vi "Find Droplets Freeze Time.vi"(8 "Error In":errorcluster, 10 "GreyLevel Drops and time Derivative in":dbl[][](array[numeric]), 11 "Rel Time Array":u32[](array[numeric])) -> (0 "Error Out":errorcluster, 3 "FreezeYesNo":T1, 4 "DropletBaselineSTD":dbl[](array[numeric]), 6 "DropletBaseline":dbl[](array[numeric]))   [LabVIEW 2013]
uses:
  TypeDef/FreezePointData.ctl
  DB/ConfDB.ctl
  DB/ConfEnum.ctl
  <vilib>/Analysis/NI_AALBase.lvlib
panel:
  out "Numeric":i32
  out "Derivative":cluster{u32[], "GreyLevelArray":dbl[]}[](graph)
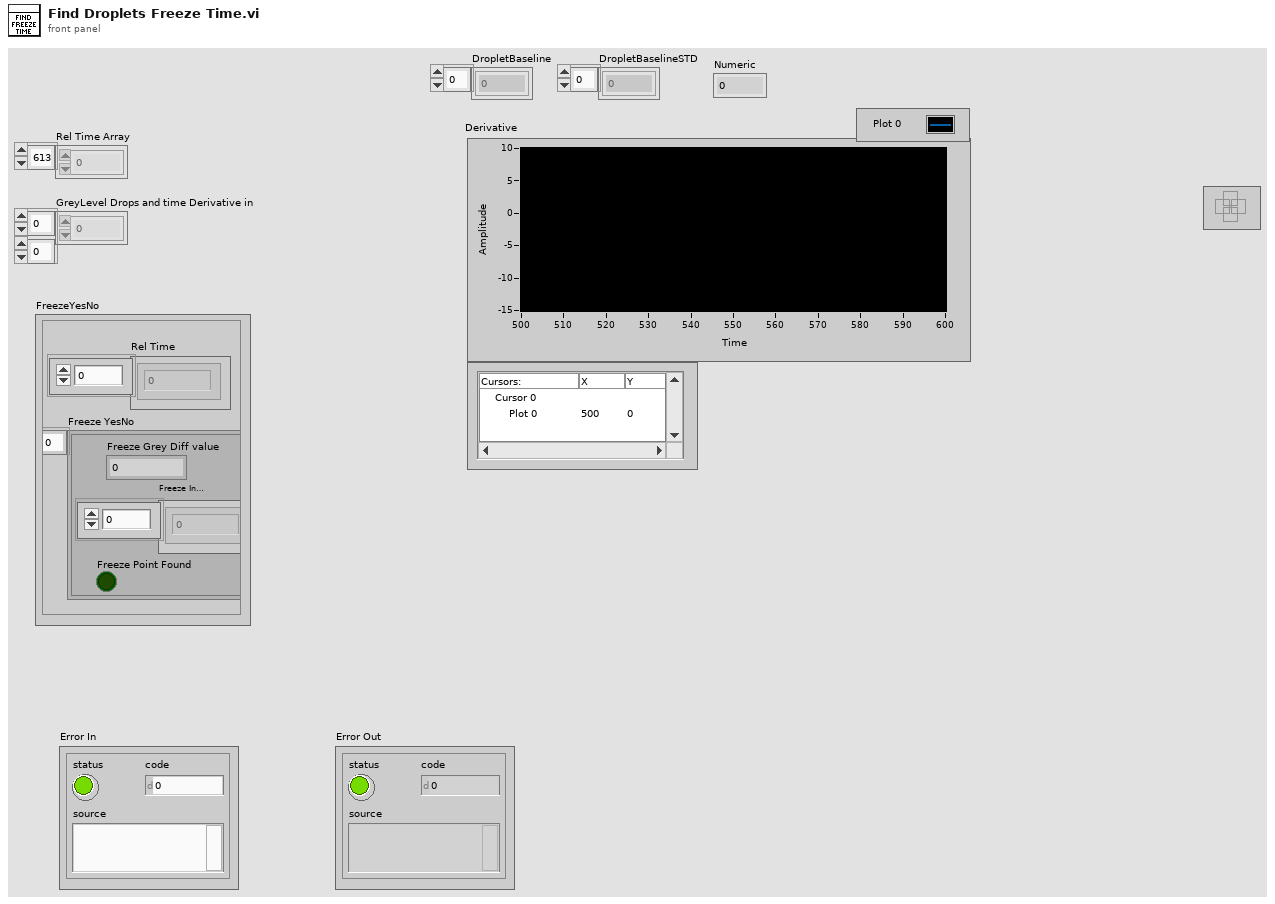
[diagram p1: front panel]
types:
  T1 = typedef "FreezePointData.ctl" = cluster{"Freeze YesNo":cluster{"Freeze Grey Diff value":dbl, "Freeze Point Found":bool, "Freeze Indices":u32[]}[], "Rel Time":u32[]}
  T2 = cluster{"Freeze Grey Diff value":dbl, "Freeze Point Found":bool, "Freeze Indices":u32[]}[]
  T3 = typedef "ConfEnum.ctl" = enum16{"Init", "GetConfDB", "GetTemperatureAtIndex", "WriteConfDB", "Configure DB"}
  T4 = typedef "ConfDB.ctl" = cluster{"NumberOfImages":i32, "NoImages2SaveAroundFreeze":i32, "Path":path, "NameOfPartialFile":string, "StartIndex":i32, "NumberOfStdTol":i32, "Detla t (sec)":i32, "Number of images for baseline":i32, "Temperature File Name":string, "Score":dbl, "Index number of Files":i32[], "End Index":i32, "Temperature Array":dbl[], "TStartIndex":i32}
  T5 = cluster{"Freeze Grey Diff value":dbl, "Freeze Point Found":bool, "Freeze Indices":u32[]}
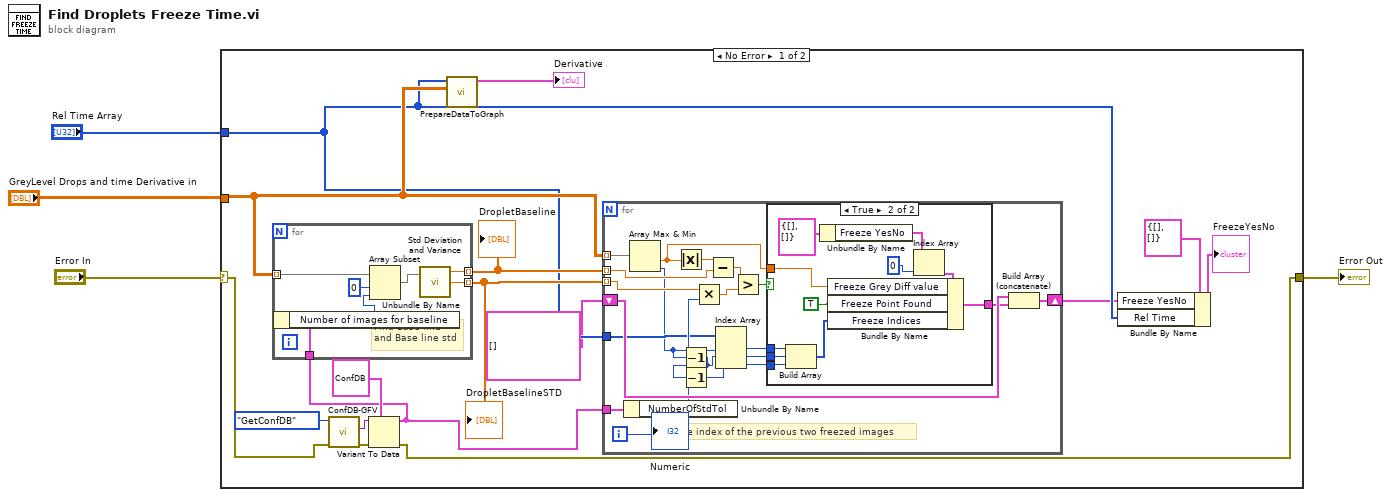
[diagram p0: block diagram]
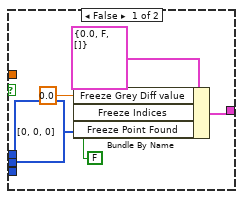
[diagram p2: hidden frame]
diagram:
  n1 = case shown="No Error" "Error In" {
    selector: "Error In" -> [w10 w65]
    tunnel: "Rel Time Array" -> [w7 _]
    tunnel: "GreyLevel Drops and time Derivative in" -> [w18 _]
    tunnel: [w9 w65] -> w1
    frame No Error {
      n2 = call "ConfDB-GFV.vi"("error in (no error)"=w10, "Command In"=ConfEnum."GetConfDB") -> ("error out"=w12:errorcluster, "Data out"=w13:variant)  [unwired: 8 in]
      n3 = Variant To Data(error in=w12, type=T4 {"NumberOfImages"=0, "NoImages2SaveAroundFreeze"=0, "Path"=path "", "NameOfPartialFile"="", "StartIndex"=0, "NumberOfStdTol"=0, "Detla t (sec)"=0, "Number of images for baseline"=0, "Temperature File Name"="", "Score"=0.0, "Index number of Files"=[], "End Index"=0, "Temperature Array"=[], "TStartIndex"=0} ("ConfDB"), Variant=w13) -> (data=w8:T4, error out=w9:errorcluster)
      n4 = for {
        tunnel: w18 -> [w58] mode=indexing
        tunnel: [w64] -> w20 mode=indexing
        tunnel: [w63] -> w19 mode=indexing
        tunnel: w8 -> [w61]
        # "Find Base line\nand Base line std"
        n5 = Unbundle By Name(w61) -> ("Number of images for baseline"=w60:i32)
        n6 = Array Subset(array=w58, index=0, length=w60) -> (w62:dbl[])
        n7 = call <vilib>:"Std Deviation and Variance.vi"("X"=w62) -> ("mean"=w64:dbl, "standard deviation"=w63:dbl)  [unwired: 1 in, 1 out]
      }
      "DropletBaseline" <- w20
      "DropletBaselineSTD" <- w19
      n8 = call "PrepareDataToGraph.vi"("GreyLevel Drops and time"=w18, "Rel Time (s)"=w7) -> ("Graph XY data"=→"Derivative":cluster{u32[], "GreyLevelArray":dbl[]}[])  [unwired: 8 in, 1 out]
      n9 = for {
        tunnel: w20 -> [w39] mode=indexing
        tunnel: w19 -> [w37] mode=indexing
        tunnel: w18 -> [w41] mode=indexing
        shift-right: [w34] -> w5
        shift-left: T2 [] -> [w33]
        tunnel: w8 -> [w31]
        tunnel: w7 -> [w29]
        i -> [w21]
        # "Find the index of the previous two freezed images"
        n10 = Unbundle By Name(w31) -> ("NumberOfStdTol"=w30:i32)
        n11 = Array Max & Min(array=w41) -> (min value=w35:dbl, min index (indices)=w27:i32)  [unwired: 2 out]
        n12 = Absolute Value(x=w35) -> (abs(x)=w40:dbl)
        n13 = Decrement(x=w27) -> (x-1=w26:i32)
        n14 = Decrement(x=w26) -> (x-1=w25:i32)
        n15 = Multiply(x=w37, y=w30) -> (x*y=w32:dbl)
        n16 = Subtract(x=w40, y=w39) -> (x-y=w38:dbl)
        n17 = Index Array(array=w29, index #1=w27, index #2=w26, index #3=w25) -> (element #1=w28:u32, element #2=w23:u32, element #3=w22:u32)
        n18 = Greater?(x=w38, y=w32) -> (0:w36:bool)
        n19 = case shown="True" w36 {
          tunnel: w28 -> [_ w51]
          tunnel: w35 -> [_ w52]
          tunnel: [w42 w53] -> w24
          tunnel: w23 -> [_ w50]
          tunnel: w22 -> [_ w49]
          frame False {
            n20 = Bundle By Name(cluster=T5 {"Freeze Grey Diff value"=0.0, "Freeze Point Found"=FALSE, "Freeze Indices"=[]} ("Min"), "Freeze Grey Diff value"=0.0 ("Minimum value"), "Freeze Indices"=u32[] [0, 0, 0], "Freeze Point Found"=FALSE ("Min Found")) -> (w42:T5)
          }
          frame True {
            n21 = Build Array(w51, w50, w49) -> (w48:u32[])
            n22 = Unbundle By Name(T1 {"Freeze YesNo"=[], "Rel Time"=[]} ("FreezeYesNo")) -> ("Freeze YesNo"=w56:T2)
            n23 = Index Array(array=w56, index=0) -> (element=w54:T5)
            n24 = Bundle By Name(cluster=w54, "Freeze Grey Diff value"=w52, "Freeze Point Found"=TRUE ("Min Found"), "Freeze Indices"=w48) -> (w53:T5)
          }
        }
        n25 = Build Array (concatenate)(w33, w24) -> (w34:T2)
        "Numeric" <- w21
      }
      n26 = Bundle By Name(cluster=T1 {"Freeze YesNo"=[], "Rel Time"=[]} ("FreezeYesNo"), "Freeze YesNo"=w5, "Rel Time"=w7) -> (→"FreezeYesNo":T1)
    }
    frame Error {
    }
  }
  "Error Out" <- w1
